vi "ND(z) at w.vi"(1 "w":dbl format="%.2f", 2 "ND(z)":dbl[](array[numeric]) format="%.2f") -> (0 "ND(w)":cdb format="%0.2f")   [LabVIEW 2020, in "NI_AALBase.lvlib"]
uses:
  <vilib>/Analysis/NI_AALBase.lvlib
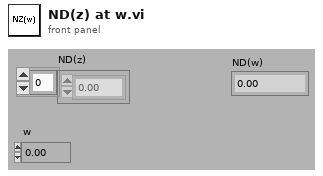
[diagram p1: front panel]
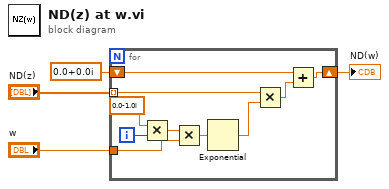
[diagram p0: block diagram]
diagram:
  n1 = for {
    shift-right: [w9] -> w1
    shift-left: cdb 0.0+0.0i -> [w7]
    tunnel: "ND(z)" -> [w6] mode=indexing
    tunnel: "w" -> [w5]
    i -> [w14]
    n2 = Multiply(x=cdb 0.0-1.0i, y=w14) -> (x*y=w12:cdb)
    n3 = Multiply(x=w12, y=w5) -> (x*y=w11:cdb)
    n4 = Exponential(1:w11) -> (0:w10:cdb)
    n5 = Multiply(x=w6, y=w10) -> (x*y=w8:cdb)
    n6 = Add(x=w7, y=w8) -> (x+y=w9:cdb)
  }
  "ND(w)" <- w1
